vi "Report Read RES Data File.vi"(8 "error in (no error)":errorcluster, 9 "template (empty)":path=path "S:/Documents/R&D Docs/Fatigue/fatigue system improvement project/HMI/Report template.xltm", 10 "Save Report Path":path=path "S:/Documents/R&D Docs/Fatigue/Fatigue results New- original" caption="selected path", 11 "RED Data File":path caption="selected path") -> (0 "error out":errorcluster)   [LabVIEW 2020]
uses:
  <vilib>/Utility/NIReport.llb/Report Type.ctl
  <vilib>/addons/_office/_exclsub.llb/font.ctl
  <vilib>/addons/_office/excel.llb/Excel Easy Table (str).vi
  <vilib>/addons/_office/excel.llb/Excel Easy Table (num).vi
  <vilib>/regexp/Match Regular Expression.xnode
  <vilib>/Utility/NIReport.llb/NI_report.lvclass
  <vilib>/Utility/NIReport.llb/NI_ReportGenerationCore.lvlib
  <vilib>/addons/_office/NI_ReportGenerationToolkit.lvlib
  <vilib>/Utility/NIReport.llb/Excel/NI_Excel.lvclass
  Report.lvlib
panel:
  out "Data":cluster{string[][]}[](array[cluster])
  out "Array 3":bool[][](array[boolean])
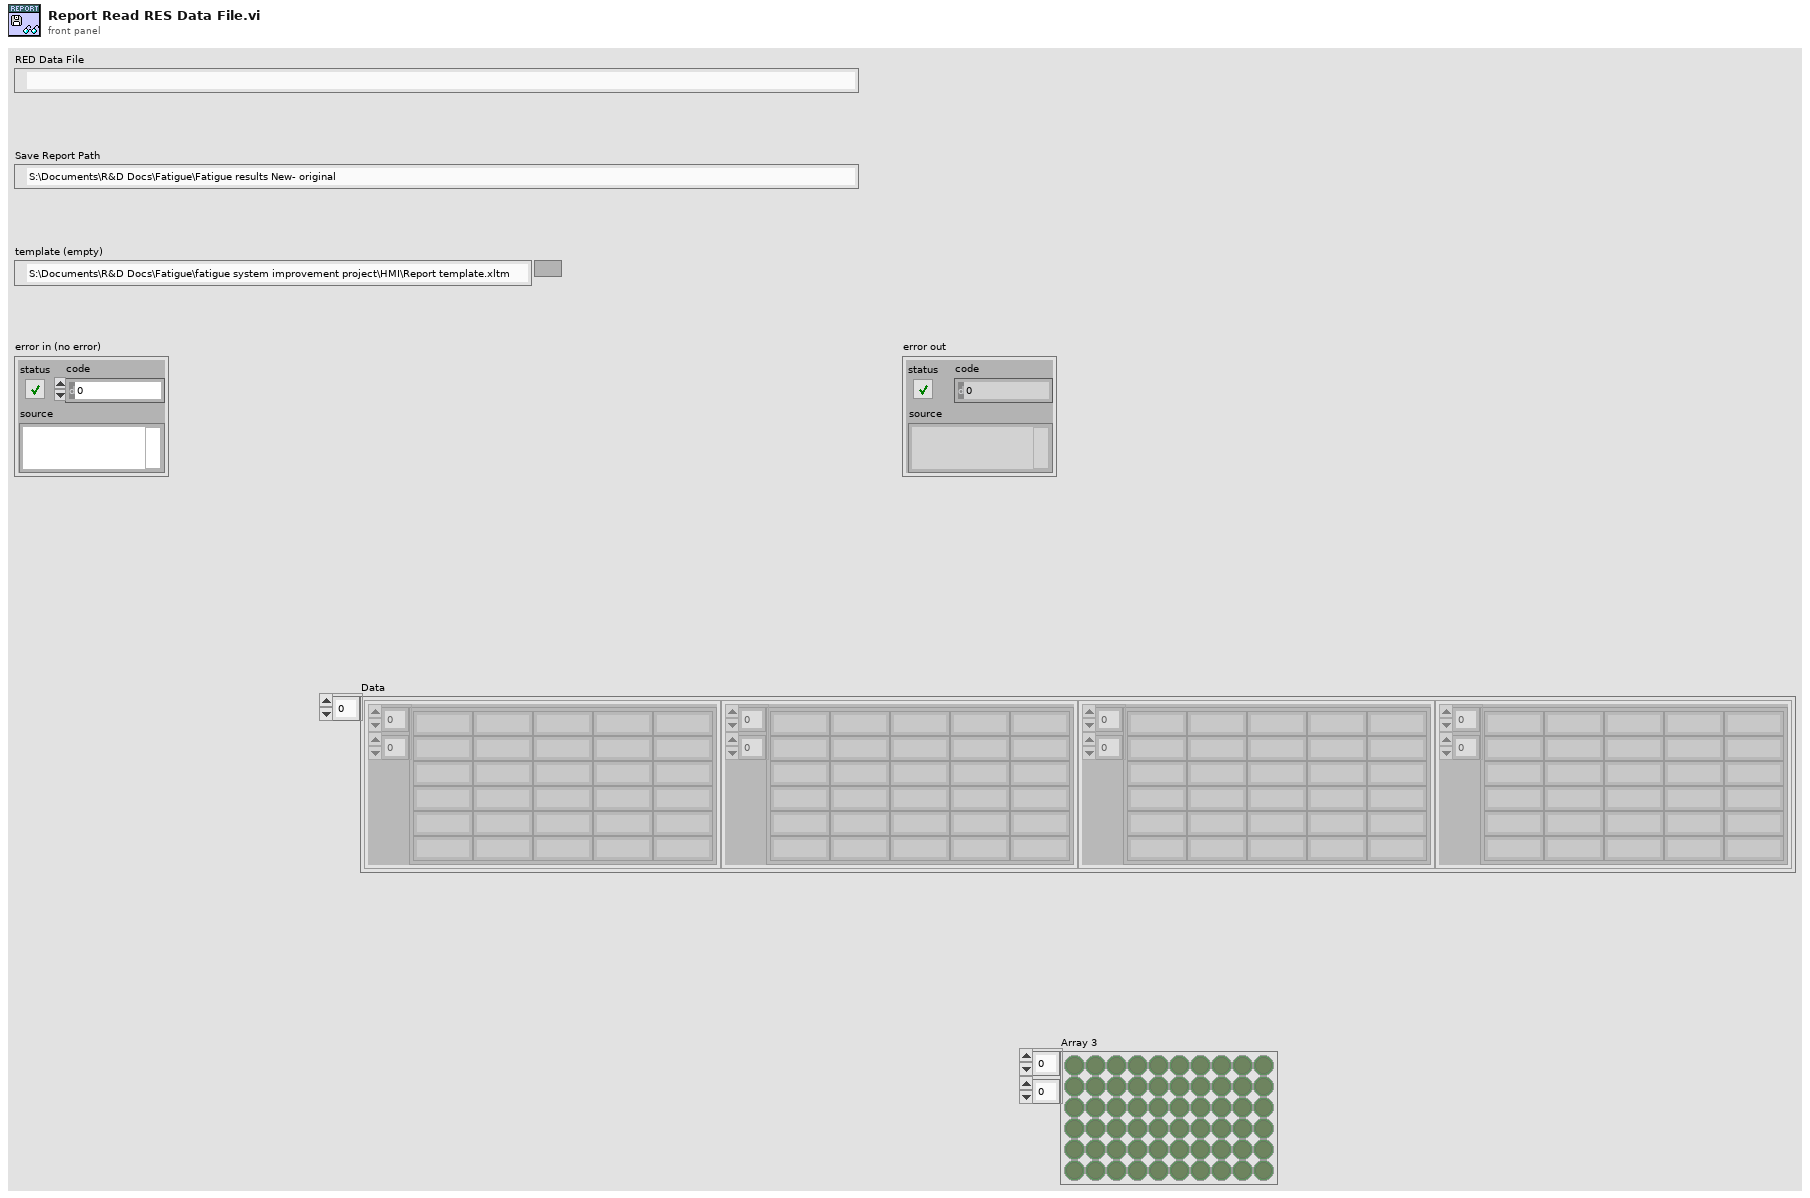
[diagram p1: front panel]
types:
  T1 = cluster{"position (excel)":cluster{"row":i32, "column":i32}, "name (excel)":string, "bookmark (word)":string}
  T2 = typedef "NI_ReportGenerationToolkit.lvlib/font.ctl" = cluster{"font name":string, "font size":dbl, "bold":u16, "italic":u16, "underline":u16, "strike through":u16, "font color":u32}
  T3 = enum16{"maximized", "minimized", "normal", "no change"}
  T4 = typedef "NI_ReportGenerationCore.lvlib/Report Type.ctl" = enum16{"HTML", "Word", "Excel"}
  T5 = enum16{"open", "open or create", "create or replace", "create", "open (read-only)"}
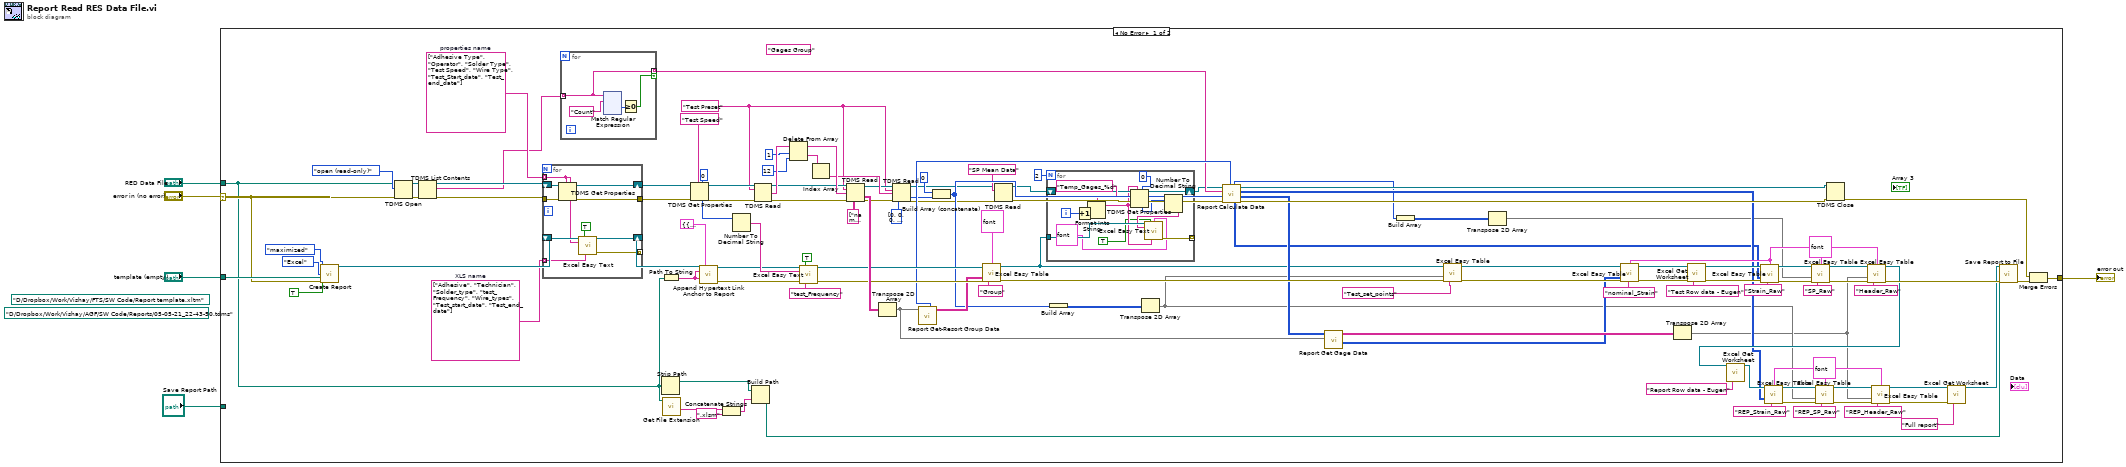
[diagram p0: block diagram]
diagram:
  (unwired) path "D:/Dropbox/Work/Vishay/FTS/SW Code/Report template.xltm" ("template (empty)")
  (unwired) path "D:/Dropbox/Work/Vishay/AGF/SW Code/Reports/05-05-21_22-43-50.tdms" ("selected path")
  n1 = case shown="No Error" "error in (no error)" {
    selector: "error in (no error)" -> [w76 w266]
    tunnel: "RED Data File" -> [w71 _]
    tunnel: "Save Report Path" -> [_ _]
    tunnel: "template (empty)" -> [w88 _]
    tunnel: [w67 w266] -> w1
    frame No Error {
      w31 = T2 {"font name"="Calibri", "font size"=11.0, "bold"=0, "italic"=0, "underline"=0, "strike through"=0, "font color"=16777216} ("font")
      (unwired) "Gages Group" ("group name")
      w43 = T2 {"font name"="Calibri", "font size"=11.0, "bold"=0, "italic"=0, "underline"=0, "strike through"=0, "font color"=16777216} ("font")
      w10 = "Test Preset" ("group name")
      w82 = string[] ["Adhesive", "Technician", "Solder_type", "test_Frequency", "Wire_types", "Test_start_date", "Test_end_date"]  # XLS name
      w117 = string[] ["Adhesive Type", "Operator", "Solder Type", "Test Speed", "Wire Type", "Test_Start_date", "Test_end_date"]  # properties name
      n2 = call <vilib>:"Create Report.vi"("window state (normal)"=T3."maximized", "display alerts? (F)"=TRUE, "report type"=Report_Type."Excel", "template (empty)"=w88, "error in (no error)"=w76) -> ("report out"=w83:refnum<class "NI_report.lvclass">)  [unwired: 9 in, 1 out]
      n3 = TDMS Open(8:w76, 10:T5."open (read-only)" ("operation"), 11:w71) -> (0:w87:errorcluster, 3:w118:refnum<k34>)  [unwired: 4 in]
      n4 = TDMS List Contents(4:w87, 7:w118) -> (0:w86:errorcluster, 2:w35:string[], 3:w116:refnum<k34>)  [unwired: 1 in, 1 out]
      n5 = for {
        tunnel: w117 -> [w264] mode=indexing
        shift-right: [w263] -> w114
        shift-left: w116 -> [w265]
        tunnel: w86 -> [w262]
        tunnel: [w261] -> w85
        shift-right: [w259] -> w81
        shift-left: w83 -> [w260]
        tunnel: w82 -> [w257] mode=indexing
        tunnel: [w255] -> _ mode=indexing
        n6 = TDMS Get Properties(5:w264, 7:w264, 8:w262, 11:w265) -> (0:w261:errorcluster, 3:w263:refnum<k34>, 4:w256:string)  [unwired: 2 in, 3 out]
        n7 = call <vilib>:"Excel Easy Text.vi"("report in"=w260, "border? (F)"=TRUE, "text"=w256, "name (\"\")"=w257) -> ("report out"=w259:refnum<class "NI_report.lvclass">, "error out"=w255:errorcluster)  [unwired: 7 in, 3 out]
      }
      n8 = for {
        tunnel: w35 -> [w138] mode=indexing
        tunnel: [w138] -> w34 mode=indexing if=w137
        n9 = xnode "Match Regular Expression"("input string"=w138, "regular expression"="Count" ("group name in (Untitled)")) -> ("offset past match"=w139:i32)  [unwired: 4 in, 4 out]
        n10 = Greater Or Equal To 0?(x=w139) -> (x >= 0?=w137:bool)
      }
      n11 = Path To String(path=w71) -> (string=w78:string)
      n12 = Strip Path(path=w71) -> (stripped path=w80:path)  [unwired: 1 out]
      n13 = call <vilib>:"Get File Extension.vi"("file"=w71) -> ("filename without extension"=w123:string)  [unwired: 6 in, 4 out]
      n14 = TDMS Get Properties(5:0, 7:"Test Speed" ("group name"), 8:w85, 11:w114) -> (0:w65:errorcluster, 3:w66:refnum<k34>, 4:w111:i32)  [unwired: 2 in, 3 out]
      n15 = call-dynamic "Append Hypertext Link Anchor to Report.vi"("report in"=w81, "MS Office parameters"=T1 {"position (excel)"={"row"=0, "column"=0}, "name (excel)"="Link_to_Row_data", "bookmark (word)"=""}, "URL of link - href"=w78, "link text"=w78) -> ("report out"=w79:refnum<class "NI_report.lvclass">, "error out"=w37:errorcluster)  [unwired: 8 in, 2 out]
      n16 = Concatenate Strings(w123, ".xlsm" ("string")) -> (w121:string)
      n17 = Number To Decimal String(number=w111) -> (decimal integer string=w110:string)  [unwired: 1 in]
      n18 = Build Path(base path=w80, name or relative path=w121) -> (appended path=w120:path)
      n19 = TDMS Read(0:w66, 5:w10, 11:w65) -> (4:w59:refnum<k34>, 8:w63:string[], 15:w64:errorcluster)  [unwired: 5 in, 3 out]
      n20 = Delete From Array(array=w63, length=1, index=12) -> (deleted portion=w58:string[], array with subset deleted=w60:string[])
      n21 = call <vilib>:"Excel Easy Text.vi"("report in"=w79, "border? (F)"=TRUE, "text"=w110, "error in (no error)"=w37, "name (\"\")"="test_Frequency" ("group name")) -> ("report out"=w105:refnum<class "NI_report.lvclass">, "error out"=w104:errorcluster)  [unwired: 6 in, 3 out]
      n22 = Index Array(array=w58) -> (element=w56:string)  [unwired: 1 in]
      n23 = TDMS Read(0:w59, 5:w10, 7:w60, 11:w64, 12:string[][] [["name", "Wire Type", "Adhesive Type", "Solder Type", "Test Speed", "Operator"]] ("property names")) -> (4:w54:refnum<k34>, 10:w106:string[][], 15:w55:errorcluster)  [unwired: 3 in, 3 out]
      n24 = Transpose 2D Array(2D array=w106) -> (transposed array=w52:string[][])
      n25 = TDMS Read(0:w54, 5:w10, 7:w56, 11:w55, 12:i32[] [0, 0, 0, 0, 0, 0] ("property names")) -> (4:w11:refnum<k34>, 10:w50:i32[], 15:w39:errorcluster)  [unwired: 3 in, 3 out]
      n26 = call "Report Get-Resort Group Data.vi"("Array in"=w52) -> ("Array 3"=w102:string[][], "Channels"=w53:i32)  [unwired: 7 in, 2 out]
      n27 = Build Array (concatenate)(0, w50) -> (w41:i32[])
      n28 = call-poly <vilib>:"Excel Easy Table.vi"("report in"=w105, "font"=T2 {"font name"="Calibri", "font size"=16.0, "bold"=0, "italic"=0, "underline"=0, "strike through"=0, "font color"=16777216}, "text data"=w102, "error in (no error)"=w104, "name (\"\")"="Group" ("name (\"\")")) -> ("report out"=w9:refnum<class "NI_report.lvclass">, "error out"=w72:errorcluster)  [unwired: 6 in, 3 out]
      n29 = TDMS Read(0:w11, 5:"SP Mean Data" ("group name in"), 11:w39) -> (4:w8:refnum<k34>, 15:w38:errorcluster)  [unwired: 5 in, 4 out]
      n30 = for {
        N: 2 -> [_]
        tunnel: w9 -> [w136]
        tunnel: [w135] -> _ mode=indexing
        shift-right: [w129] -> w6
        shift-left: w8 -> [w132]
        i -> [w127]
        n31 = Increment(x=w127) -> (x+1=w126:i32)
        n32 = Format Into String(format string="Temp_Gages_%d" ("group name"), w126) -> (resulting string=w128:string)  [unwired: 2 in, 1 out]
        n33 = TDMS Get Properties(5:0, 7:w128, 11:w132) -> (3:w129:refnum<k34>, 4:w131:i32)  [unwired: 3 in, 4 out]
        n34 = Number To Decimal String(number=w131) -> (decimal integer string=w130:string)  [unwired: 1 in]
        n35 = call <vilib>:"Excel Easy Text.vi"("report in"=w136, "border? (F)"=TRUE, "font"=T2 {"font name"="Calibri", "font size"=11.0, "bold"=0, "italic"=0, "underline"=0, "strike through"=0, "font color"=16777216}, "text"=w130, "name (\"\")"=w128) -> ("error out"=w135:errorcluster)  [unwired: 6 in, 4 out]
      }
      n36 = Build Array(w41) -> (w100:i32[][])
      n37 = Transpose 2D Array(2D array=w100) -> (transposed array=w21:i32[][])
      n38 = call "Report Calculate Data.vi"("Channels #"=w53, "error in (no error)"=w38, "Report SP"=w41, "Group Names"=w34, "Refnum in"=w6) -> ("error out"=w70:errorcluster, "Max Array Report"=w51:i32[][], "Mean Array Report"=w22:i32[][], "Refnum out"=w98:refnum<k34>, "Mean Array"=w19:i32[][], "ALL Points"=w17:i32[])  [unwired: 1 out]
      n39 = call "Report Get Gage Data.vi"("Gage Data"=w52, "Array"=w51) -> ("Array 2"=w44:i32[][], "Array 3"=w90:string[][])  [unwired: 7 in, 1 out]
      n40 = Build Array(w17) -> (w18:i32[][])
      n41 = call-poly <vilib>:"Excel Easy Table.vi"("report in"=w9, "text data"=w21, "error in (no error)"=w72, "name (\"\")"="Test_set_points" ("name (\"\")")) -> ("report out"=w49:refnum<class "NI_report.lvclass">, "error out"=w46:errorcluster)  [unwired: 7 in, 3 out]
      n42 = Transpose 2D Array(2D array=w18) -> (transposed array=w16:i32[][])
      n43 = call-poly <vilib>:"Excel Easy Table.vi"("report in"=w49, "font"=w43, "text data"=w44, "error in (no error)"=w46, "name (\"\")"="nominal_Strain" ("name (\"\")")) -> ("report out"=w48:refnum<class "NI_report.lvclass">, "error out"=w45:errorcluster)  [unwired: 6 in, 3 out]
      n44 = Transpose 2D Array(2D array=w90) -> (transposed array=w20:string[][])
      n45 = call <vilib>:"Excel Get Worksheet.vi"("report in"=w48, "error in (no error)"=w45, "name (\"\")"="Test Row data - Eugen" ("name (\"\")")) -> ("report out"=w96:refnum<class "NI_report.lvclass">, "error out"=w75:errorcluster)  [unwired: 11 in]
      n46 = call-poly <vilib>:"Excel Easy Table.vi"("report in"=w96, "font"=w43, "text data"=w19, "error in (no error)"=w75, "name (\"\")"="Strain_Raw" ("name (\"\")")) -> ("report out"=w94:refnum<class "NI_report.lvclass">, "error out"=w93:errorcluster)  [unwired: 6 in, 3 out]
      n47 = call-poly <vilib>:"Excel Easy Table.vi"("report in"=w94, "font"=w43, "text data"=w16, "error in (no error)"=w93, "name (\"\")"="SP_Raw" ("name (\"\")")) -> ("report out"=w92:refnum<class "NI_report.lvclass">, "error out"=w74:errorcluster)  [unwired: 6 in, 3 out]
      n48 = TDMS Close(8:w70, 11:w98) -> (0:w68:errorcluster)  [unwired: 1 out]
      n49 = call-poly <vilib>:"Excel Easy Table.vi"("report in"=w92, "font"=w43, "text data"=w20, "error in (no error)"=w74, "name (\"\")"="Header_Raw" ("name (\"\")")) -> ("report out"=w32:refnum<class "NI_report.lvclass">, "error out"=w73:errorcluster)  [unwired: 6 in, 3 out]
      n50 = call <vilib>:"Excel Get Worksheet.vi"("report in"=w32, "name (\"\")"="Report Row data - Eugen" ("name (\"\")")) -> ("report out"=w23:refnum<class "NI_report.lvclass">)  [unwired: 12 in, 1 out]
      n51 = call-poly <vilib>:"Excel Easy Table.vi"("report in"=w23, "font"=w31, "text data"=w22, "name (\"\")"="REP_Strain_Raw" ("name (\"\")")) -> ("report out"=w25:refnum<class "NI_report.lvclass">, "error out"=w26:errorcluster)  [unwired: 7 in, 3 out]
      n52 = call-poly <vilib>:"Excel Easy Table.vi"("report in"=w25, "font"=w31, "text data"=w21, "error in (no error)"=w26, "name (\"\")"="REP_SP_Raw" ("name (\"\")")) -> ("report out"=w27:refnum<class "NI_report.lvclass">, "error out"=w30:errorcluster)  [unwired: 6 in, 3 out]
      n53 = call-poly <vilib>:"Excel Easy Table.vi"("report in"=w27, "font"=w31, "text data"=w20, "error in (no error)"=w30, "name (\"\")"="REP_Header_Raw" ("name (\"\")")) -> ("report out"=w15:refnum<class "NI_report.lvclass">, "error out"=w12:errorcluster)  [unwired: 6 in, 3 out]
      n54 = call <vilib>:"Excel Get Worksheet.vi"("report in"=w15, "error in (no error)"=w12, "name (\"\")"="Full report" ("name (\"\")")) -> ("report out"=w13:refnum<class "NI_report.lvclass">)  [unwired: 11 in, 1 out]
      n55 = call-dynamic "Save Report to File.vi"("report in"=w13, "report file path"=w120, "error in (no error)"=w73) -> ("error out"=w69:errorcluster)  [unwired: 11 in, 1 out]
      n56 = Merge Errors(w68, w69) -> (w67:errorcluster)
    }
    frame Error {
    }
  }
  "error out" <- w1
